vi "RemoveSlashes.vi"(10 "slashed string":string) -> (2 "unslashed":string)   [LabVIEW 2014, in "Raspberry Pi Compatible Compiler for LabVIEW.lvlib" / "Python Functions.lvlib"]
uses:
  Python Functions.lvlib
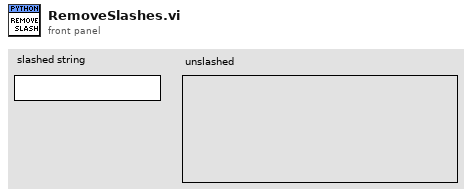
[diagram p1: front panel]
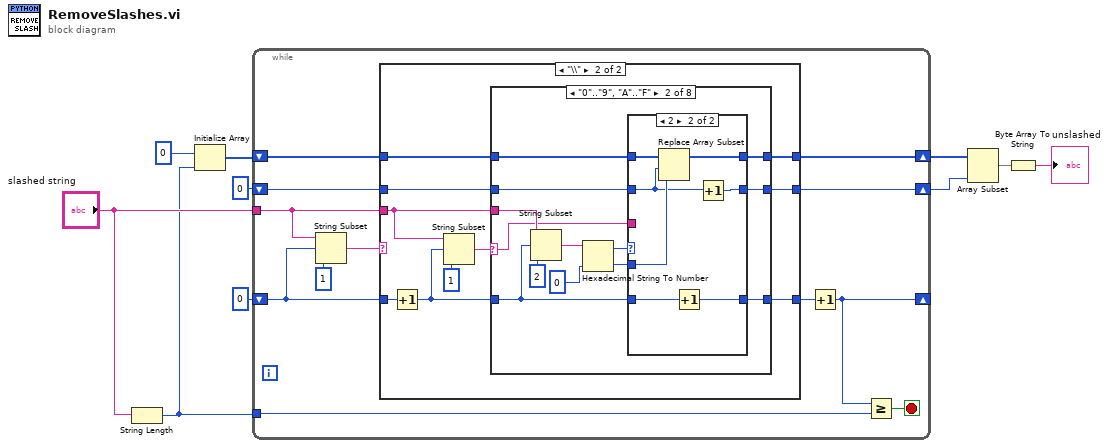
[diagram p0: block diagram]
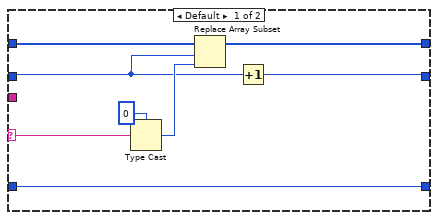
[diagram p2: hidden frame]
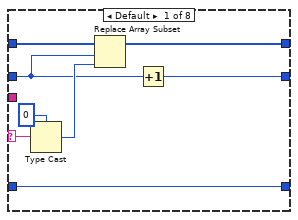
[diagram p3: hidden frame]
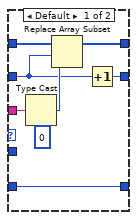
[diagram p4: hidden frame]
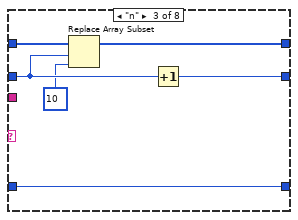
[diagram p5: hidden frame]
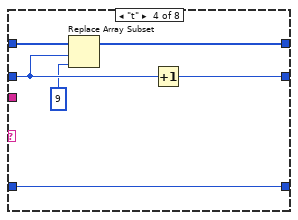
[diagram p6: hidden frame]
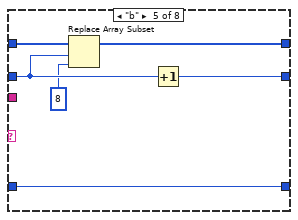
[diagram p7: hidden frame]
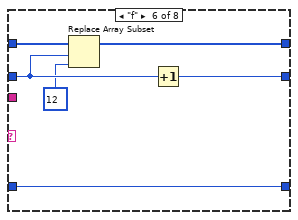
[diagram p8: hidden frame]
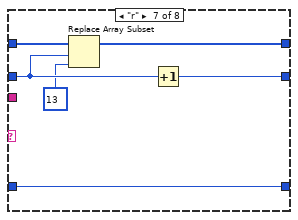
[diagram p9: hidden frame]
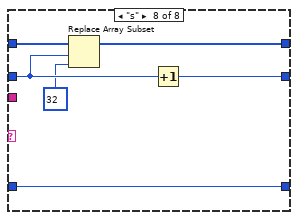
[diagram p10: hidden frame]
diagram:
  n1 = String Length(string="slashed string") -> (length=w1:i32)
  n2 = Initialize Array(u8 0 ("element"), w1) -> (w10:u8[])
  n3 = while {
    tunnel: "slashed string" -> [w19]
    shift-right: [w15] -> w6
    shift-left: w10 -> [w20]
    shift-right: [w12] -> _
    shift-left: 0 -> [w18]
    shift-right: [w16] -> w5
    shift-left: 0 -> [w17]
    tunnel: w1 -> [w11]
    stop <- w13 stop-if-true
    n4 = String Subset(string=w19, offset (0)=w18, length (rest)=1 ("length (rest)")) -> (substring=w21:string)
    n5 = case shown="\"\\\\\"" w21 {
      selector: w21 -> [w26 _]
      tunnel: w20 -> [w28 w38]
      tunnel: w19 -> [_ w31]
      tunnel: w18 -> [w23 w39]
      tunnel: w17 -> [w25 w35]
      tunnel: [w24 w34] -> w16
      tunnel: [w27 w33] -> w15
      tunnel: [w23 w32] -> w14
      frame Default {
        n6 = Type Cast(type=u8 0, x=w26) -> (*(type *) &x=w29:u8)
        n7 = Replace Array Subset(array=w28, new element=w29, index=w25) -> (w27:u8[])
        n8 = Increment(x=w25) -> (x+1=w24:i32)
      }
      frame "\\" {
        n9 = Increment(x=w39) -> (x+1=w36:i32)
        n10 = String Subset(string=w31, offset (0)=w36, length (rest)=1 ("length (rest)")) -> (substring=w37:string)
        n11 = case shown="\"0\"..\"9\", \"A\"..\"F\"" w37 {
          selector: w37 -> [w48 w49 _ _ _ _ _ _]
          tunnel: w38 -> [w46 w56 w82 w88 w94 w100 w106 w112]
          tunnel: w36 -> [w41 w52 w77 w83 w89 w95 w101 w107]
          tunnel: w35 -> [w43 w54 w81 w87 w93 w99 w105 w111]
          tunnel: [w42 w53 w80 w86 w92 w98 w104 w110] -> w34
          tunnel: [w45 w55 w78 w84 w90 w96 w102 w108] -> w33
          tunnel: [w41 w50 w77 w83 w89 w95 w101 w107] -> w32
          tunnel: w31 -> [_ w51 _ _ _ _ _ _]
          frame Default {
            n12 = Type Cast(type=u8 0, x=w48) -> (*(type *) &x=w44:u8)
            n13 = Replace Array Subset(array=w46, new element=w44, index=w43) -> (w45:u8[])
            n14 = Increment(x=w43) -> (x+1=w42:i32)
          }
          frame "0".."9", "A".."F" {
            n15 = String Subset(string=w51, offset (0)=w52, length (rest)=2 ("length (rest)")) -> (substring=w60:string)
            n16 = Hexadecimal String To Number(string=w60, default (0uL)=u8 0 ("default (0 U32)")) -> (offset past number=w58:i32, number=w57:u8)  [unwired: 1 in]
            n17 = case shown="2" w58 {
              tunnel: w57 -> [_ w74]
              tunnel: w56 -> [w64 w76]
              tunnel: [w63 w75] -> w55
              tunnel: w54 -> [w65 w73]
              tunnel: [w62 w72] -> w53
              tunnel: w52 -> [w69 w71]
              tunnel: w49 -> [w67 _]
              tunnel: [w69 w70] -> w50
              frame Default {
                n18 = Type Cast(type=u8 0, x=w67) -> (*(type *) &x=w66:u8)
                n19 = Replace Array Subset(array=w64, new element=w66, index=w65) -> (w63:u8[])
                n20 = Increment(x=w65) -> (x+1=w62:i32)
              }
              frame 2 {
                n21 = Replace Array Subset(array=w76, new element=w74, index=w73) -> (w75:u8[])
                n22 = Increment(x=w71) -> (x+1=w70:i32)
                n23 = Increment(x=w73) -> (x+1=w72:i32)
              }
            }
          }
          frame "n" {
            n24 = Replace Array Subset(array=w82, new element=u8 10 ("new element/subarray"), index=w81) -> (w78:u8[])
            n25 = Increment(x=w81) -> (x+1=w80:i32)
          }
          frame "t" {
            n26 = Replace Array Subset(array=w88, new element=u8 9 ("new element/subarray"), index=w87) -> (w84:u8[])
            n27 = Increment(x=w87) -> (x+1=w86:i32)
          }
          frame "b" {
            n28 = Replace Array Subset(array=w94, new element=u8 8 ("new element/subarray"), index=w93) -> (w90:u8[])
            n29 = Increment(x=w93) -> (x+1=w92:i32)
          }
          frame "f" {
            n30 = Replace Array Subset(array=w100, new element=u8 12 ("new element/subarray"), index=w99) -> (w96:u8[])
            n31 = Increment(x=w99) -> (x+1=w98:i32)
          }
          frame "r" {
            n32 = Replace Array Subset(array=w106, new element=u8 13 ("new element/subarray"), index=w105) -> (w102:u8[])
            n33 = Increment(x=w105) -> (x+1=w104:i32)
          }
          frame "s" {
            n34 = Replace Array Subset(array=w112, new element=u8 32 ("new element/subarray"), index=w111) -> (w108:u8[])
            n35 = Increment(x=w111) -> (x+1=w110:i32)
          }
        }
      }
    }
    n36 = Increment(x=w14) -> (x+1=w12:i32)
    n37 = Greater Or Equal?(x=w12, y=w11) -> (x >= y?=w13:bool)
  }
  n38 = Array Subset(array=w6, length=w5) -> (w4:u8[])  [unwired: 1 in]
  n39 = Byte Array To String(unsigned byte array=w4) -> (string=→"unslashed":string)
